vi "Projeto_Modbus_Finalizado.vi"() -> ()   [LabVIEW 2016]
panel:
  out "ThetaPlace":i16
  out "ThetaPick":i16
  out "PlaceY":i16
  out "PlaceX":i16
  out "PickY":i16
  out "PickX":i16
  in  "My_Turn":bool
  out "Confirma_Sinal":bool
  out "Game_Over":bool
  out "Passa_Vez":bool
  out "Dobrao":bool
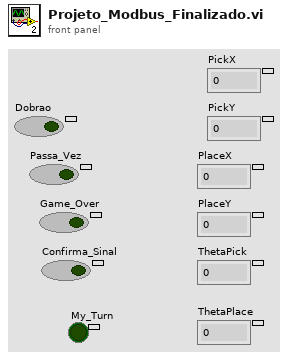
[diagram p1: front panel]
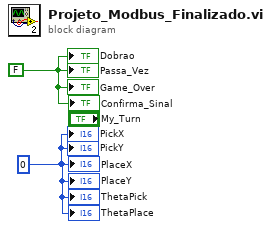
[diagram p0: block diagram]
diagram:
  w1 = FALSE ("Passa_Vez")
  w2 = i16 0 ("PlaceX")
  "Dobrao" <- w1
  "Passa_Vez" <- w1
  "Game_Over" <- w1
  "Confirma_Sinal" <- w1
  "PickX" <- w2
  "PickY" <- w2
  "PlaceX" <- w2
  "PlaceY" <- w2
  "ThetaPick" <- w2
  "ThetaPlace" <- w2
